vi "XIPIN_3GPP_Turbo_Decoder_4_0.vi"   [LabVIEW 2017]
doc: "Discontinued. Please select the 3GPP Mixed Mode Turbo Decoder. The Turbo Decoder LogiCORE from Xilinx is a high-performance, compact Turbo Decoder which meets the 3GPP specification. The core is delivered through the Xilinx CORE Generator System and integrates seamlessly with the Xilinx design flow.\n------------------------------------\n<b>Need License</b> : Yes"
uses:
  <vilib>/rvi/XilinxIP/XIPIN_XNode/niFpgaXIPIN.xnode
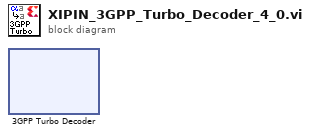
[diagram p0: block diagram]
diagram:
  n1 = xnode ("3GPP Turbo Decoder")() -> ()
